vi "OE1311&OE1351_Configure Sine Out.vi"(7 "OE1300_Configure Sine Out":T1={"Sine Output Amplitude (V)"=0.1, "SineOut Mode"=0} {"SineOut Mode" items=["OFF", "Fixed"]; "Sine Output Amplitude (V)" min=0.0001 max=5.0 format="%#.4g"}, 8 "Error in (no error)":errorcluster caption="error out（no error）", 9 "Remote Mode":u16(ring)=1 items=["RS232"=1, "Ethernet"=3], 10 "Connection ID in":refnum<k5>, 11 "VISA resource name":refnum<visa-resource-name>) -> (0 "Error out":errorcluster caption="error out", 1 "Output String":string, 2 "Connection ID out":refnum<k5>, 3 "VISA resource  out":refnum<visa-resource-name>)   [LabVIEW 2011]
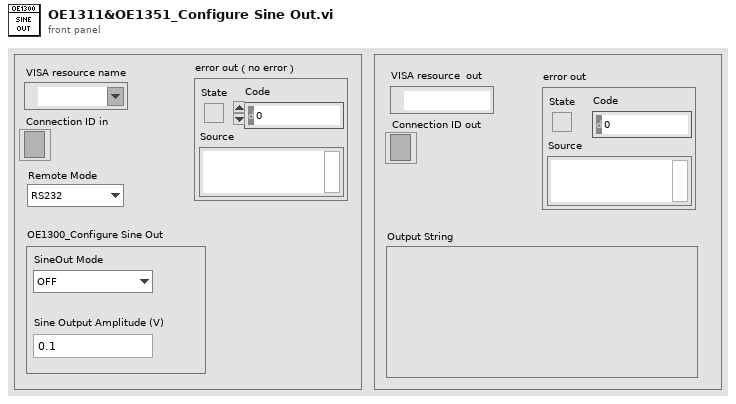
[diagram p1: front panel]
types:
  T1 = cluster{"Sine Output Amplitude (V)":dbl, "SineOut Mode":u8}
  T2 = enum16{"ISRC", "IGND", "ICPL", "ILIN", "PHAS", "FMOD", "RSLP", "FREQ", "SWPT", "SLLM", "SULM", "SSLL", "SSLG", "STLM", "SWRM", "IRNG", "SENS", "RMOD", "OFLT", "OFSL", "SYNC", "DMOD", "HARM", "DARB", "SWVT", "SLVL", "SVLL", "SVUL", "SVSL", "SVSG", "SVTM", "SVRM", "RALL", "SNAP", "OUTP", "OAUX", "COUT", "CAUX", "COFP", "CEXP", "FPOP", "OEXP", "*IDN", "*RST", "OVLD", "INOV", "GNOV", "*PLL", "SSET", "RSET", "AGAN", "APHS", "ARSV", "ASCL", "EQCD", "EQCS", "SPED", "SRAT", "SLEN", "SSLE", "STRG", "SPRM", "STRD", "PAUS", "REST", "SPTS", "TRCA", "TEMP", "RSTU", "IHNZ", "DEQU", "SADD", "ARNG", "CSPE", "ISRCD", "IGNDD", "ICPLD", "ILIND", "PHASD", "FMODD", "RSLPD", "FREQD", "SWPTD", "SLLMD", "SULMD", "SSLLD", "SSLGD", "STLMD", "SWRMD", "SENSD", "RMODD", "OFLTD", "OFSLD", "SYNCD", "HARMD", "EQCDD", "EQCSD", "SNAPD", "OUTPD", "SWVTD", "SLVLD", "SVLLD", "SVULD", "SVSLD", "SVSGD", "SVTMD", "SVRMD", "SVDCD", "ARSVD", "AGAND", "APHSD", "ASCLD", "FPOPD", "CAUXD", "OEXPD", "SPEDD", "SRATD", "SLEND", "SSLED", "STRGD", "SPRMD", "STRDD", "PAUSD", "RESTD", "SPTSD", "TRCAD", "*IDND", "*RSTD", "INOVD", "GNOVD", "*PLLD", "SSETD", "RSETD", "RALLD"}
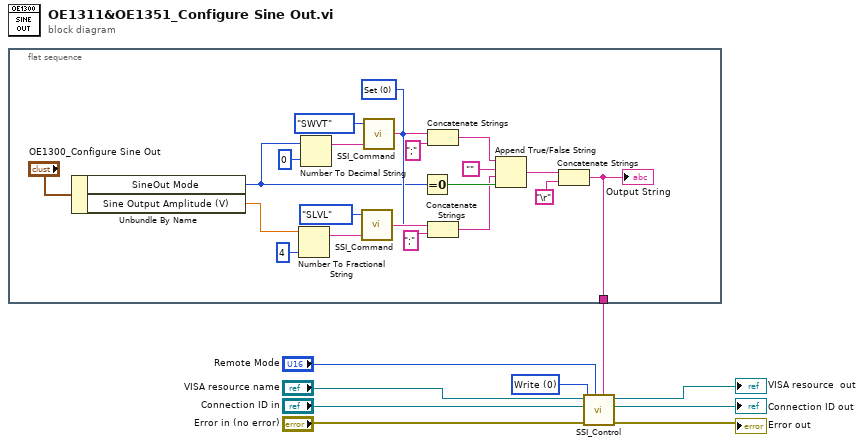
[diagram p0: block diagram]
diagram:
  w7 = u16 0 items=["Write", "Read"] ("Control")
  n1 = flat-sequence {
    tunnel: [w24] -> w1
    frame #0 {
      w18 = u16 0 items=["Set", "Query"] ("Opera")
      n2 = Unbundle By Name("OE1300_Configure Sine Out") -> ("SineOut Mode"=w13:u8, "Sine Output Amplitude (V)"=w17:dbl)
      n3 = Number To Fractional String(number=w17, precision (6)=i16 4 ("宽度(-)")) -> (F-format string=w28:string)  [unwired: 2 in]
      n4 = Number To Decimal String(number=w13, width (-)=i16 0 ("宽度(-)")) -> (decimal integer string=w22:string)
      n5 = call "SSI_Command.vi"("Opera"=w18, "Paramter"=w28, "Command Type"=T2."SLVL") -> ("Output string"=w27:string)  [unwired: 1 in]
      n6 = call "SSI_Command.vi"("Opera"=w18, "Paramter"=w22, "Command Type"=T2."SWVT") -> ("Output string"=w20:string)  [unwired: 1 in]
      n7 = Equal To 0?(x=w13) -> (x = 0?=w14:bool)
      n8 = Concatenate Strings(w20, ";" ("替换字符串(\"\")")) -> (w12:string)
      n9 = Concatenate Strings(w27, ";" ("替换字符串(\"\")")) -> (w10:string)
      n10 = Append True/False String(1:w14, 2:w10, 3:"", 4:w12) -> (0:w15:string)
      n11 = Concatenate Strings(w15, "\r") -> (w24:string)
      "Output String" <- w24
    }
  }
  n12 = call "SSI_Control.vi"("Write Buffer"=w1, "Remote Mode"="Remote Mode", "Error in (no error)"="Error in (no error)", "Control"=w7, "Connection ID in"="Connection ID in", "VISA resource name"="VISA resource name") -> ("Error out"=→"Error out":errorcluster, "Connection ID out"=→"Connection ID out":refnum<k5>, "VISA resource  out"=→"VISA resource  out":refnum<visa-resource-name>)  [unwired: 2 in, 1 out]
